vi "c_ctre_phoenix6_serialize_bool.vi"(0 "Numeric 2":i32, 1 "Numeric 3":u8, 2 "String 2":string) -> (20 "Numeric":i32, 21 "String":string)   [LabVIEW 2023]
uses:
  <vilib>/Rock Robotics/WPI/ThirdParty/Phoenix-LabVIEW/Controls/DriverLib.ctl
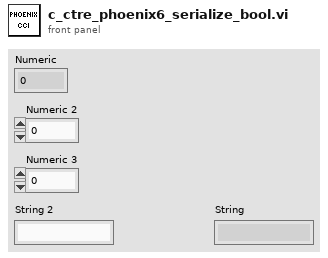
[diagram p1: front panel]
types:
  T1 = typedef "DriverLib.ctl" = path
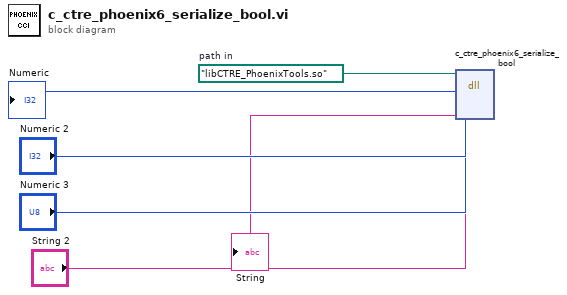
[diagram p0: block diagram]
diagram:
  w6 = T1 path "libCTRE_PhoenixTools.so"  # path in
  n1 = dll-call lib="?" fn="c_ctre_phoenix6_serialize_bool"(path in=w6, "Numeric 2", "Numeric 3", "String 2") -> (→"Numeric":i32, →"String":string)  [unwired: 4 in, 2 out]
